vi "make_stage_array (SubVI).vi"(11 "Stage settings:":T1={"Set stage?"=FALSE, "start X (um)"=0.0, "stop X (um) "=0.0, "# X Steps"=1, "start Y (um)"=0.0, "stop Y (um) "=0.0, "# Y steps"=1, "start Z (um)"=0.0, "stop Z (um)"=0.0, "# Z steps "=1, "Sweep?"=FALSE, "Dir to sweep"=0, "Amplitude (um)"=0.0, "Frequency (Hz)"=41.0} {"Dir to sweep" items=["X", "Y", "Z"]}) -> (3 "Tot Stage Arr":dbl[][](array[numeric]))   [LabVIEW 2014]
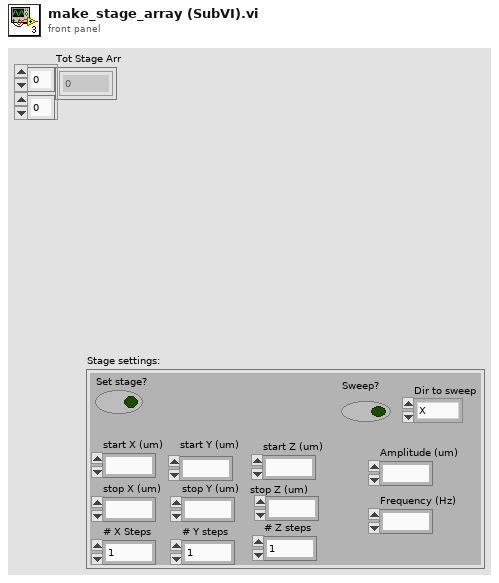
[diagram p1: front panel]
types:
  T1 = cluster{"Set stage?":bool, "start X (um)":ext, "stop X (um) ":ext, "# X Steps":i32, "start Y (um)":ext, "stop Y (um) ":ext, "# Y steps":i32, "start Z (um)":ext, "stop Z (um)":ext, "# Z steps ":i32, "Sweep?":bool, "Dir to sweep":u16, "Amplitude (um)":ext, "Frequency (Hz)":ext}
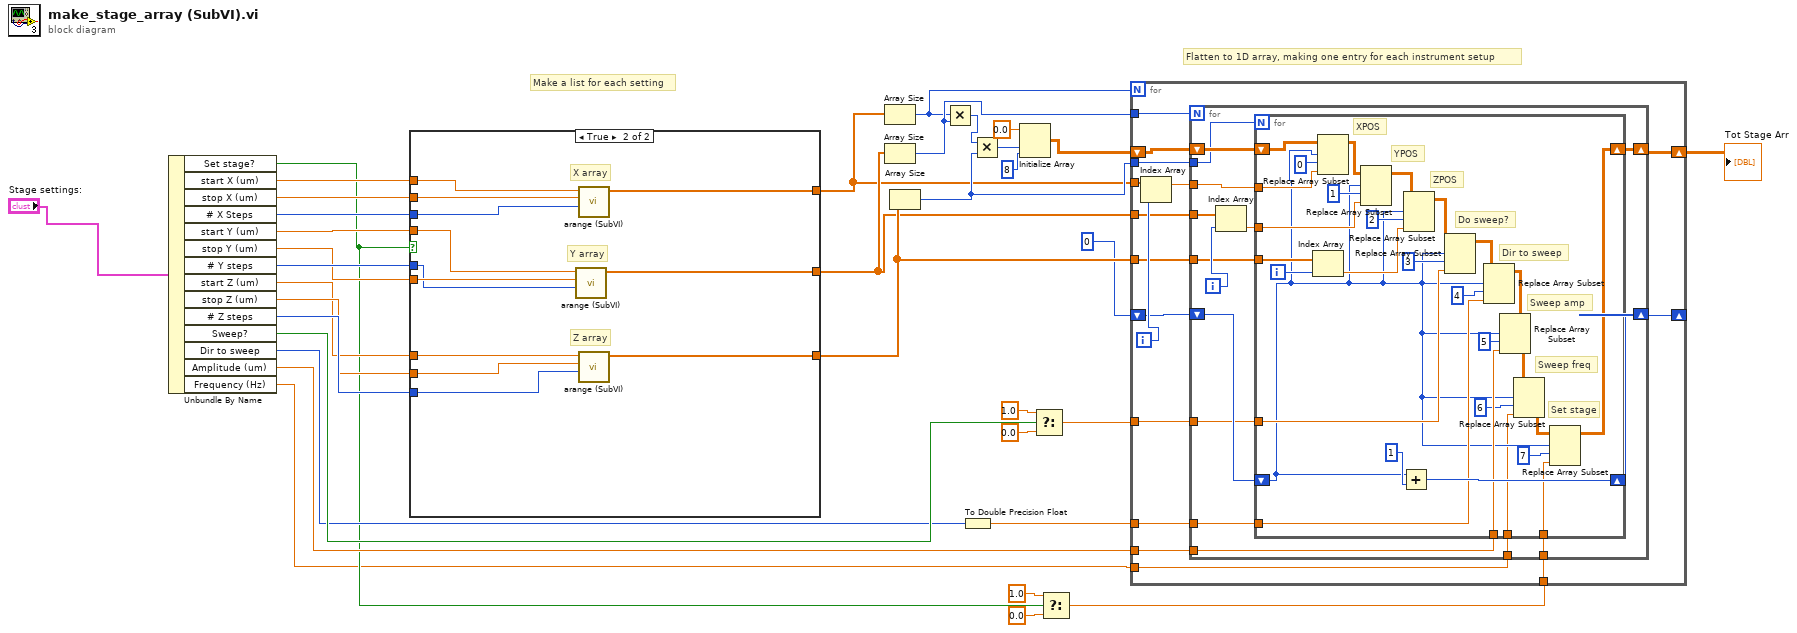
[diagram p0: block diagram]
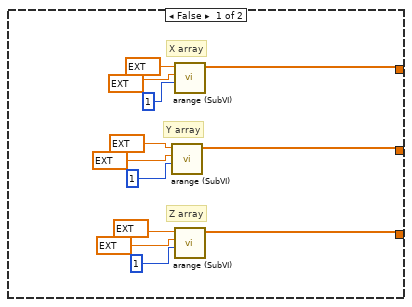
[diagram p2: hidden frame]
diagram:
  # "Make a list for each setting"
  # "Flatten to 1D array, making one entry for each instrument setup"
  n1 = Unbundle By Name("Stage settings:") -> ("Set stage?"=w3:bool, "start X (um)"=w14:ext, "stop X (um)"=w15:ext, "# X Steps"=w16:i32, "start Y (um)"=w17:ext, "stop Y (um)"=w18:ext, "# Y steps"=w19:i32, "start Z (um)"=w20:ext, "stop Z (um)"=w21:ext, "# Z steps"=w22:i32, "Sweep?"=w12:bool, "Dir to sweep"=w8:u16, "Amplitude (um)"=w6:ext, "Frequency (Hz)"=w1:ext)
  n2 = case shown="True" w3 {
    tunnel: w14 -> [_ w59]
    tunnel: w15 -> [_ w58]
    tunnel: w16 -> [_ w57]
    tunnel: w17 -> [_ w56]
    tunnel: w18 -> [_ w55]
    tunnel: w19 -> [_ w54]
    tunnel: w20 -> [_ w53]
    tunnel: w21 -> [_ w52]
    tunnel: w22 -> [_ w51]
    tunnel: [w38 w50] -> w30
    tunnel: [w37 w49] -> w31
    tunnel: [w36 w48] -> w32
    frame False {
      # "Z array"
      # "Y array"
      # "X array"
      n3 = call "arange (SubVI).vi"("# Steps"=1, "stop"=ext -9999.0, "start"=ext -9999.0) -> ("Array"=w37:ext[])  [unwired: 8 in]
      n4 = call "arange (SubVI).vi"("# Steps"=1, "stop"=ext -9999.0, "start"=ext -9999.0) -> ("Array"=w38:ext[])  [unwired: 8 in]
      n5 = call "arange (SubVI).vi"("# Steps"=1, "stop"=ext -9999.0, "start"=ext -9999.0) -> ("Array"=w36:ext[])  [unwired: 8 in]
    }
    frame True {
      # "Z array"
      # "Y array"
      # "X array"
      n6 = call "arange (SubVI).vi"("# Steps"=w54, "stop"=w55, "start"=w56) -> ("Array"=w49:ext[])  [unwired: 8 in]
      n7 = call "arange (SubVI).vi"("# Steps"=w57, "stop"=w58, "start"=w59) -> ("Array"=w50:ext[])  [unwired: 8 in]
      n8 = call "arange (SubVI).vi"("# Steps"=w51, "stop"=w52, "start"=w53) -> ("Array"=w48:ext[])  [unwired: 8 in]
    }
  }
  n9 = Array Size(array=w30) -> (size(s)=w33:i32)
  n10 = Array Size(array=w31) -> (size(s)=w34:i32)
  n11 = Array Size(array=w32) -> (size(s)=w35:i32)
  n12 = Multiply(x=w33, y=w34) -> (x*y=w24:i32)
  n13 = To Double Precision Float(number=w8) -> (double precision float=w7:dbl)
  n14 = Multiply(x=w24, y=w35) -> (x*y=w25:i32)
  n15 = Initialize Array(0.0 ("element"), w25, 8 ("dimension size")) -> (w27:dbl[][])
  n16 = Select(t=1.0, s=w12, f=0.0) -> (s? t:f=w9:dbl)
  n17 = Select(t=1.0, s=w3, f=0.0) -> (s? t:f=w2:dbl)
  n18 = for {
    N: w33 -> [_]
    shift-right: [w65] -> _
    shift-left: 0 ("disabled index (row)") -> [w66]
    shift-right: [w74] -> w29
    shift-left: w27 -> [w75]
    tunnel: w30 -> [w73]
    tunnel: w31 -> [w70]
    tunnel: w32 -> [w69]
    tunnel: w34 -> [w68]
    tunnel: w35 -> [w67]
    tunnel: w9 -> [w64]
    tunnel: w7 -> [w63]
    tunnel: w6 -> [w62]
    tunnel: w2 -> [w61]
    tunnel: w1 -> [w60]
    i -> [w71]
    n19 = Index Array(array=w73, index=w71) -> (element=w72:ext)
    n20 = for {
      N: w68 -> [_]
      tunnel: w72 -> [w88]
      tunnel: w70 -> [w87]
      tunnel: w69 -> [w84]
      tunnel: w67 -> [w83]
      shift-right: [w89] -> w74
      shift-left: w75 -> [w90]
      shift-right: [w81] -> w65
      shift-left: w66 -> [w82]
      tunnel: w64 -> [w80]
      tunnel: w63 -> [w79]
      tunnel: w62 -> [w78]
      tunnel: w61 -> [w77]
      tunnel: w60 -> [w76]
      i -> [w86]
      n21 = Index Array(array=w87, index=w86) -> (element=w85:ext)
      n22 = for {
        N: w83 -> [_]
        tunnel: w88 -> [w114]
        tunnel: w85 -> [w113]
        tunnel: w84 -> [w111]
        shift-right: [w93] -> w89
        shift-left: w90 -> [w120]
        shift-right: [w108] -> w81
        shift-left: w82 -> [w95]
        tunnel: w80 -> [w105]
        tunnel: w79 -> [w102]
        tunnel: w78 -> [w99]
        tunnel: w77 -> [w92]
        tunnel: w76 -> [w91]
        i -> [w112]
        # "Set stage"
        # "Sweep freq"
        # "Sweep amp"
        # "Dir to sweep"
        # "Do sweep?"
        # "ZPOS"
        # "YPOS"
        # "XPOS"
        n23 = Index Array(array=w111, index=w112) -> (element=w110:ext)
        n24 = Replace Array Subset(array=w120, new element=w114, index (row)=w95, index (col)=0 ("disabled index (col)")) -> (w118:dbl[][])
        n25 = Replace Array Subset(array=w118, new element=w113, index (row)=w95, index (col)=1 ("disabled index (col)")) -> (w117:dbl[][])
        n26 = Add(x=w95, y=1) -> (x+y=w108:i32)
        n27 = Replace Array Subset(array=w117, new element=w110, index (row)=w95, index (col)=2 ("disabled index (col)")) -> (w107:dbl[][])
        n28 = Replace Array Subset(array=w107, new element=w105, index (row)=w95, index (col)=3 ("disabled index (col)")) -> (w104:dbl[][])
        n29 = Replace Array Subset(array=w104, new element=w102, index (row)=w95, index (col)=4 ("disabled index (col)")) -> (w101:dbl[][])
        n30 = Replace Array Subset(array=w101, new element=w99, index (row)=w95, index (col)=5 ("disabled index (col)")) -> (w98:dbl[][])
        n31 = Replace Array Subset(array=w98, new element=w91, index (row)=w95, index (col)=6 ("disabled index (col)")) -> (w96:dbl[][])
        n32 = Replace Array Subset(array=w96, new element=w92, index (row)=w95, index (col)=7 ("disabled index (col)")) -> (w93:dbl[][])
      }
    }
  }
  "Tot Stage Arr" <- w29
